vi "Query Condition Status.vi"(0 "VISA resource name":refnum<visa-resource-name>, 11 "error in (no error)":errorcluster) -> (4 "VISA resource name out":refnum<visa-resource-name>, 6 "Condition":i32 format="%.0x", 15 "error out":errorcluster)   [LabVIEW 2013, in "Yokogawa PZ4000.lvlib"]
doc: "This VI reads the Condition Register from the PZ4000 series."
uses:
  <instrlib>/Yokogawa PZ4000/Yokogawa PZ4000.lvlib
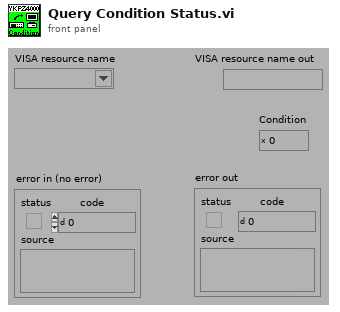
[diagram p1: front panel]
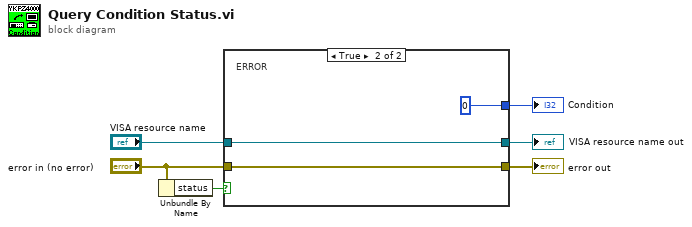
[diagram p0: block diagram]
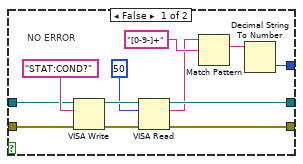
[diagram p2: hidden frame]
diagram:
  n1 = Unbundle By Name("error in (no error)") -> ("status"=w2:bool)
  n2 = case shown="True" w2 {
    tunnel: "VISA resource name" -> [w11 w19]
    tunnel: "error in (no error)" -> [w14 w21]
    tunnel: [w16 0] -> w5
    tunnel: [w12 w21] -> w4
    tunnel: [w9 w19] -> w1
    frame False {
      # "NO ERROR"
      n3 = VISA Write(VISA resource name=w11, write buffer="STAT:COND?", error in (no error)=w14) -> (VISA resource name out=w10:refnum<visa-resource-name>, error out=w13:errorcluster)  [unwired: 1 out]
      n4 = VISA Read(VISA resource name=w10, byte count=u32 50, error in (no error)=w13) -> (VISA resource name out=w9:refnum<visa-resource-name>, read buffer=w7:string, error out=w12:errorcluster)  [unwired: 1 out]
      n5 = Match Pattern(string=w7, regular expression="[0-9-]+") -> (match substring=w17:string)  [unwired: 1 in, 3 out]
      n6 = Decimal String To Number(string=w17) -> (number=w16:i32)  [unwired: 2 in, 1 out]
    }
    frame True {
      # "ERROR"
    }
  }
  "error out" <- w4
  "Condition" <- w5
  "VISA resource name out" <- w1
